vi "MGI ERD Base Factory.vi"(10 "error":errorcluster, 11 "MGI Error Reporter Dialog in":refnum<class "MGI Error Reporter Dialog.lvclass">) -> (2 "MGI ERD LB Row Base":refnum<class "MGI ERD LB Row Base.lvclass">)   [LabVIEW 2016, in "MGI Error Reporter Dialog.lvclass"]
doc: "This dynamic dispatch VI selects the appropriate ERD Base Class for the specified error. A Child class may override this VI, which always uses the MGI ERD LB Row Time and Count.lvclass\n\nAuthored by Shawn Walpole\nsupport@mooregoodideas.com\nwww.mooregoodideas.com\n\nCopyright (c) 2013, Moore Good Ideas, Inc.\n\nAll rights reserved.\n\nRedistribution and use in source and binary forms, with or without modification, are permitted provided that the following conditions are met:\n\n * Redistributions of source code must retain the above copyright notice, this list of conditions and the following disclaimer.\n * Redistributions in binary form must reproduce the above copyright notice, this list of conditions and the following disclaimer in the documentation and/or other materials provided with the distribution.\n * Neither the name of Moore Good Ideas, Inc. nor the names of its contributors may be used to endorse or promote products derived from this software without specific prior written permission.\n\nTHIS SOFTWARE IS PROVIDED BY THE COPYRIGHT HOLDERS AND CONTRIBUTORS \"AS IS\" AND ANY EXPRESS OR IMPLIED WARRANTIES, INCLUDING, BUT NOT LIMITED TO, THE IMPLIED WARRANTIES OF MERCHANTABILITY AND FITNESS FOR A PARTICULAR PURPOSE ARE DISCLAIMED. IN NO EVENT SHALL THE COPYRIGHT OWNER OR CONTRIBUTORS BE LIABLE FOR ANY DIRECT, INDIRECT, INCIDENTAL, SPECIAL, EXEMPLARY, OR CONSEQUENTIAL DAMAGES (INCLUDING, BUT NOT LIMITED TO, PROCUREMENT OF SUBSTITUTE GOODS OR SERVICES; LOSS OF USE, DATA, OR PROFITS; OR BUSINESS INTERRUPTION) HOWEVER CAUSED AND ON ANY THEORY OF LIABILITY, WHETHER IN CONTRACT, STRICT LIABILITY, OR TORT (INCLUDING NEGLIGENCE OR OTHERWISE) ARISING IN ANY WAY OUT OF THE USE OF THIS SOFTWARE, EVEN IF ADVISED OF THE POSSIBILITY OF SUCH DAMAGE."
uses:
  <userlib>/_MGI/Error Reporter/MGI Error Reporter Dialog/MGI Error Reporter Dialog.lvclass
  <userlib>/_MGI/Error Reporter/MGI Error Reporter Dialog/MGI ERD LB Row Base/MGI ERD LB Row Base.lvclass
  <userlib>/_MGI/Error Reporter/MGI Error Reporter Dialog/MGI ERD LB Row Time and Count/MGI ERD LB Row Time and Count.lvclass
  C:/Program Files (x86)/National Instruments/LabVIEW 2016/user.lib/_MGI/Error Reporter/MGI Error Reporter Dialog/MGI ERD LB Row Base/MGI ERD LB Row Base.lvclass
panel:
  out "MGI ERD LB Row Time and Count in":refnum<class "MGI ERD LB Row Time and Count.lvclass">
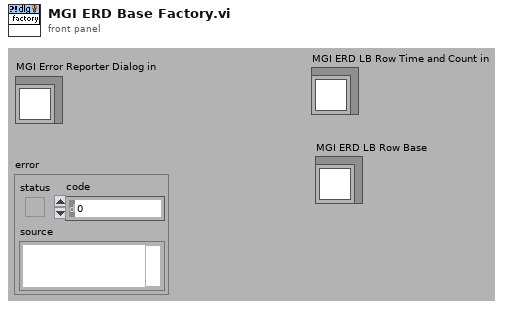
[diagram p1: front panel]
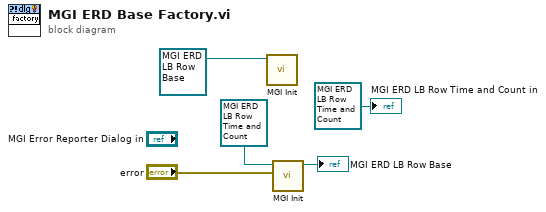
[diagram p0: block diagram]
diagram:
  n1 = call-dynamic "MGI Init.vi"("MGI ERD LB Row Base in"=refnum<class "MGI ERD LB Row Base.lvclass"> refnum ("MGI ERD LB Row Base")) -> ()  [unwired: 1 in, 10 out]
  n2 = call-dynamic "MGI Init.vi"("error"="error", "MGI ERD LB Row Time and Count in"=refnum<class "MGI ERD LB Row Time and Count.lvclass"> refnum) -> ("MGI ERD LB Row Time and Count out"=→"MGI ERD LB Row Base":refnum<class "MGI ERD LB Row Time and Count.lvclass">)  [unwired: 9 out]
  "MGI ERD LB Row Time and Count in" <- refnum<class "MGI ERD LB Row Time and Count.lvclass"> refnum ("MGI ERD LB Row Time and Count in")
